vi "Add Scale.vi"(8 "error in (no error)":errorcluster, 11 "references":T1) -> (0 "error out":errorcluster)   [LabVIEW 2013, in "Scaling editor node.lvclass"]
uses:
  Scaling editor node.lvclass
  <vilib>/NI/DCAF Table API/Table Manager/object ref.ctl
  <vilib>/NI/Tag Bus Data Framework/Configuration Editor/Classes/Engine Parent/Engine Parent Editor Node.lvclass
  <vilib>/NI/Tag Bus Data Framework/Configuration Editor/Classes/Module editor node/module editor node.lvclass
  module/configuration/Scaling configuration.lvclass
  Scaling editor node.lvclass/Scaling editor node.ctl
  <vilib>/NI/DCAF Table API/Table Manager/Table Manager.lvclass
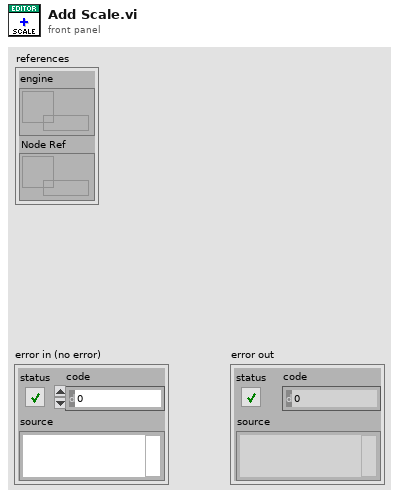
[diagram p1: front panel]
types:
  T1 = typedef "Table Manager.lvlib/Table Manager.lvclass/object ref.ctl" = cluster{"engine":refnum<data-value>, "Node Ref":refnum<data-value>}
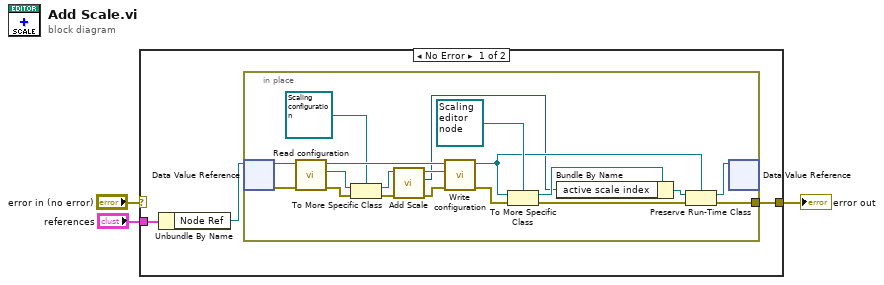
[diagram p0: block diagram]
diagram:
  n1 = case shown="No Error" "error in (no error)" {
    selector: "error in (no error)" -> [_ w26]
    tunnel: [w6 w26] -> w2
    tunnel: "references" -> [w4 _]
    frame No Error {
      n2 = Unbundle By Name(w4) -> ("Node Ref"=w5:refnum<data-value>)
      n3 = in-place {
        in-place-border: [w13] -> w6
        n4 = in-place-dvr #1(w5) -> (w24:refnum<class "module editor node.lvclass">, w22:errorcluster)
        n5 = call-dynamic "Read configuration.vi"("error in"=w22, "NISE_CEF_serializable node in"=w24) -> ("error out"=w20:errorcluster, "configuration"=w23:refnum<class "NISE_CEF_serializable configuration.lvclass">, "NISE_CEF_serializable node out"=w25:refnum<class "module editor node.lvclass">)  [unwired: 7 in]
        n6 = To More Specific Class(target class=refnum<class "Scaling configuration.lvclass"> refnum ("Scaling configuration"), reference=w23, error in=w20) -> (specific class reference=w16:refnum<class "Scaling configuration.lvclass">, error out=w19:errorcluster)
        n7 = call-dynamic "Add Scale.vi"("error in (no error)"=w19, "Scaling configuration in"=w16) -> ("error out"=w18:errorcluster, "new index"=w7:i32, "Scaling configuration out"=w17:refnum<class "Scaling configuration.lvclass">)  [unwired: 7 in]
        n8 = call-dynamic "Write configuration.vi"("error in"=w18, "configuration"=w17, "NISE_CEF_serializable node in"=w25) -> ("error out"=w15:errorcluster, "NISE_CEF_serializable node out"=w11:refnum<class "module editor node.lvclass">)  [unwired: 7 in]
        n9 = To More Specific Class(target class=refnum<class "Scaling editor node.lvclass"> refnum ("Scaling editor node"), reference=w11, error in=w15) -> (specific class reference=w9:refnum<class "Scaling editor node.lvclass">, error out=w10:errorcluster)
        n10 = Bundle By Name(cluster=w9, "active scale index"=w7) -> (w8:refnum<class "Scaling editor node.lvclass">)
        n11 = Preserve Run-Time Class(object in=w8, error in=w10, 2:w11) -> (object out=w12:refnum<class "module editor node.lvclass">, error out=w13:errorcluster)
        n12 = in-place-dvr #1(w12) -> ()  [unwired: 2 out]
      }
    }
    frame Error {
    }
  }
  "error out" <- w2
